vi "285_Initialize_1.vi"(8 "error in (no error)":errorcluster caption="错误输入（无错误）") -> (0 "错误输出":errorcluster, 3 "VISA资源名称输出":refnum<visa-resource-name>)   [LabVIEW 2018]
uses:
  <vilib>/Instr/_visa.llb/VISA Configure Serial Port (Instr).vi
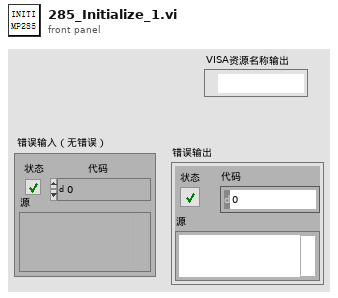
[diagram p1: front panel]
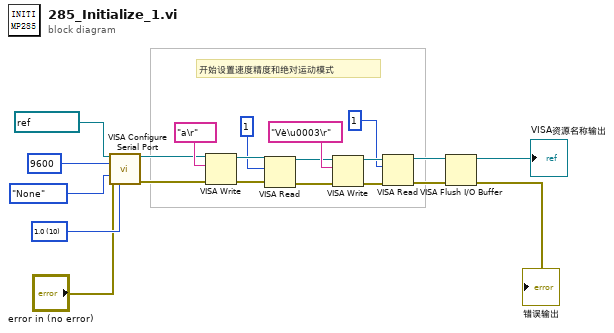
[diagram p0: block diagram]
diagram:
  w4 = u16 10 items=["1.0"=10, "1.5"=15, "2.0"=20] ("停止位 (10: 1位)")
  # "开始设置速度精度和绝对运动模式"
  n1 = call-poly "VISA Configure Serial Port"("VISA resource name"=refnum<visa-resource-name> "COM8" ("VISA资源名称"), "baud rate (9600)"=u32 9600 ("波特率(9600)"), "parity (0:none)"=enum16{"None", "Odd", "Even", "Mark", "Space"}."None" ("校验（无）"), "error in (no error)"="error in (no error)", "stop bits (10: 1 bit)"=w4) -> ("VISA resource name out"=w11:refnum<visa-resource-name>, "error out"=w10:errorcluster)  [unwired: 9 in]
  n2 = VISA Write ("VISA写入")(VISA resource name=w11, write buffer="a\r" ("写入缓冲区"), error in (no error)=w10) -> (VISA resource name out=w18:refnum<visa-resource-name>, error out=w19:errorcluster)  [unwired: 1 out]
  n3 = VISA Read(VISA resource name=w18, byte count=u32 1 ("字节总数"), error in (no error)=w19) -> (VISA resource name out=w17:refnum<visa-resource-name>, error out=w16:errorcluster)  [unwired: 2 out]
  n4 = VISA Write ("VISA写入")(VISA resource name=w17, write buffer="Vè\u0003\r" ("写入缓冲区"), error in (no error)=w16) -> (VISA resource name out=w13:refnum<visa-resource-name>, error out=w14:errorcluster)  [unwired: 1 out]
  n5 = VISA Read(VISA resource name=w13, byte count=u32 1 ("字节总数"), error in (no error)=w14) -> (VISA resource name out=w8:refnum<visa-resource-name>, error out=w9:errorcluster)  [unwired: 2 out]
  n6 = VISA Flush I/O Buffer(VISA resource name=w8, error in (no error)=w9) -> (VISA resource name out=→"VISA资源名称输出":refnum<visa-resource-name>, error out=→"错误输出":errorcluster)  [unwired: 1 in]
